vi "GenerateSquare.vi"(11 "CA":T1(array[cluster])) -> (0 "New square":T2, 2 "Match":bool, 3 "updated CA":T1(array[cluster]))   [LabVIEW 2020]
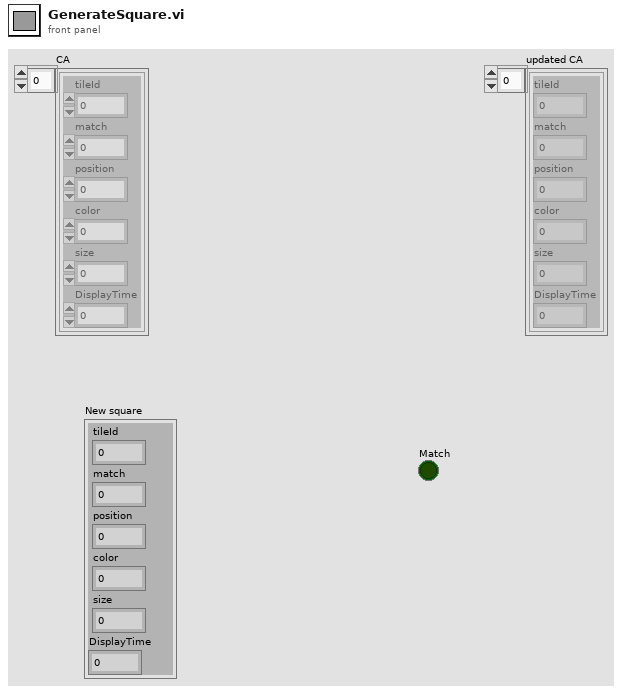
[diagram p1: front panel]
types:
  T1 = cluster{"tileId":i32, "match":i32, "position":i32, "color":u32, "size":i32, "DisplayTime":i32}[]
  T2 = cluster{"tileId":i32, "match":i32, "position":i32, "color":u32, "size":i32, "DisplayTime":i32}
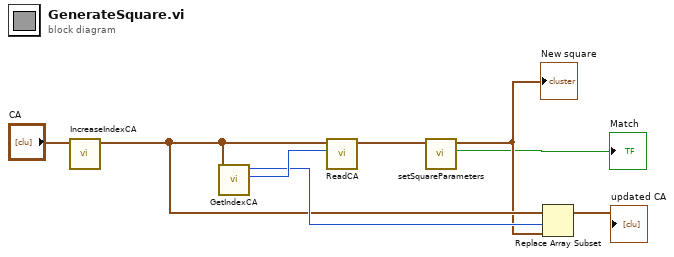
[diagram p0: block diagram]
diagram:
  n1 = call "IncreaseIndexCA.vi"("CA"="CA") -> ("updatedCA"=w5:T1)  [unwired: 10 in]
  n2 = call "GetIndexCA.vi"("CA"=w5) -> ("N-index"=w8:i32, "Current index"=w6:u8)  [unwired: 9 in]
  n3 = call "ReadCA.vi"("CA"=w5, "Index"=w8) -> ("square"=w7:T2)  [unwired: 8 in]
  n4 = call "setSquareParameters.vi"("square in"=w7) -> ("Match"=→"Match":bool, "square out"=w4:T2)  [unwired: 9 in]
  "New square" <- w4
  n5 = Replace Array Subset(array=w5, new element=w4, index=w6) -> (→"updated CA":T1)
